vi "RT Main.vi"() -> ()   [LabVIEW 2015]
doc: "The myRIO Custom FPGA Project template acquires button data from the onboard button and displays the button value on a Boolean indicator. The SYS.RDY indicator shows the FPGA status."
uses:
  <vilib>/rvi/interface/nirviOpenFPGA/nirviOpenFPGA.xnode
  <vilib>/rvi/interface/nirviReadWriteControl/nirviReadWriteControl.xnode
  <vilib>/rvi/interface/nirviCloseFPGA/nirviCloseFPGA.xnode
  NiFpgaLv.dll
  <vilib>/Utility/error.llb/Error Cluster From Error Code.vi
  <vilib>/rvi/interface/Simulation/niFpgaSimulationCallBeginRW.vi
  <vilib>/rvi/errors/niLvFpgaAdjustHostInterfaceError.vi
  <vilib>/Utility/error.llb/DialogType.ctl
  <vilib>/FPGAPlugInAG/Dynamic/niLvFpga_Close_Dynamic.vi
  FPGA Bitfiles/DCServo_FPGATarget_ParallaxStandard_7tCb1f0l5I8.lvbitx
  Parallax Standard Servo (FPGA).vi
  <vilib>/FPGAPlugInAG/myRIO-1900/niLvFpga_Open_myRIO-1900.vi
  <vilib>/rvi/interface/common/dynamic/niFpgaDynamicAddResources.vi
  <vilib>/userdefined/High Color/nirio_resource_hc.ctl
panel:
  in  "servo_0_ccw angle":dbl(knob) scale=0.0..180.0
  in  "servo_0_ccw offset":fxp<+/-,32,4>
  in  "resource name":T1
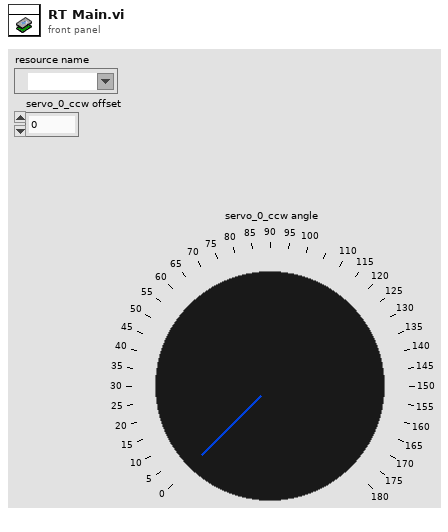
[diagram p1: front panel]
types:
  T1 = typedef "nirio_resource_hc.ctl" = tag
  T2 = typedef "DialogType.ctl" = u16
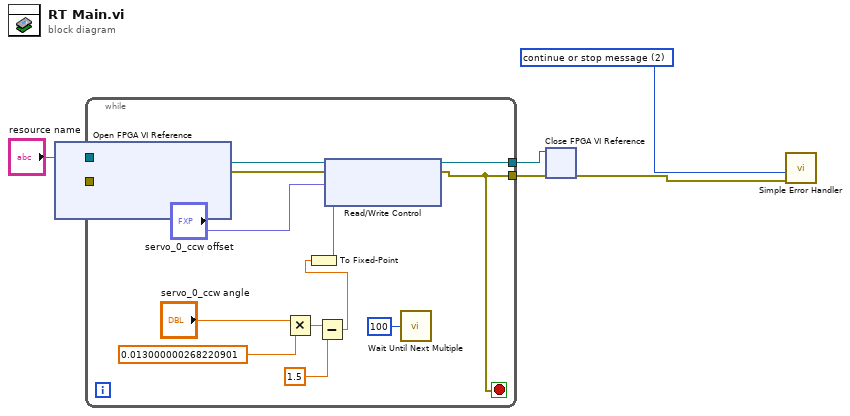
[diagram p0: block diagram]
diagram:
  w2 = T2 2 items=["no dialog", "OK message", "continue or stop message", "OK message + warnings", "continue/stop + warnings"] ("type of dialog (OK msg:1)")
  n1 = xnode "Open FPGA VI Reference"("resource name"="resource name") -> ("FPGA VI Reference Out"=w7:refnum<k20>, "error out"=w6:errorcluster)  [unwired: 1 in]
  n2 = while {
    tunnel: w7 -> [w19]
    tunnel: w6 -> [w18]
    tunnel: [w15] -> w4
    tunnel: [w14] -> w1
    stop <- w15 stop-if-true
    n3 = Multiply(x="servo_0_ccw angle", y=0.013000000268220901) -> (x*y=w11:dbl)
    n4 = Subtract(x=w11, y=1.5) -> (x-y=w8:dbl)
    n5 = To Fixed-Point(number=w8) -> (fixed-point=w9:fxp<+/-,32,16>)  [unwired: 1 in]
    n6 = xnode "Read/Write Control"("FPGA VI Reference In"=w19, "error in"=w18, "servo_0_ccw offset"="servo_0_ccw offset", "servo_0_ccw angle"=w9) -> ("FPGA VI Reference Out"=w14:refnum<k20>, "error out"=w15:errorcluster)
    n7 = call "Wait Until Next Multiple"("Count(mSec)"=u32 100) -> ()  [unwired: 1 out]
  }
  n8 = xnode "Close FPGA VI Reference"("FPGA VI Reference In"=w1, "error in"=w4) -> ("error out"=w3:errorcluster)
  n9 = call <vilib>:"Simple Error Handler.vi"("type of dialog (OK msg:1)"=w2, "error in (no error)"=w3) -> ()  [unwired: 3 in, 5 out]
